vi "取像框架 - 複製.vi"() -> ()   [LabVIEW 2015]
uses:
  <vilib>/userdefined/High Color/IMAQdx.ctl
  <vilib>/vision/driver/NI_Vision_Acquisition_Software.lvlib
  <vilib>/vision/NI_Vision_Development_Module.lvlib
panel:
  in  "開圖":bool
  in  "影像數量":i32=1
  in  "Slide":i16(slide) min=0 scale=0.0..2.0
  in  "Session In":T1="cam1"
  in  "重新開圖":bool
  in  "取像":bool
  out "error out":errorcluster
  in  "stop":bool
  out "Image":T2(plugin-control)
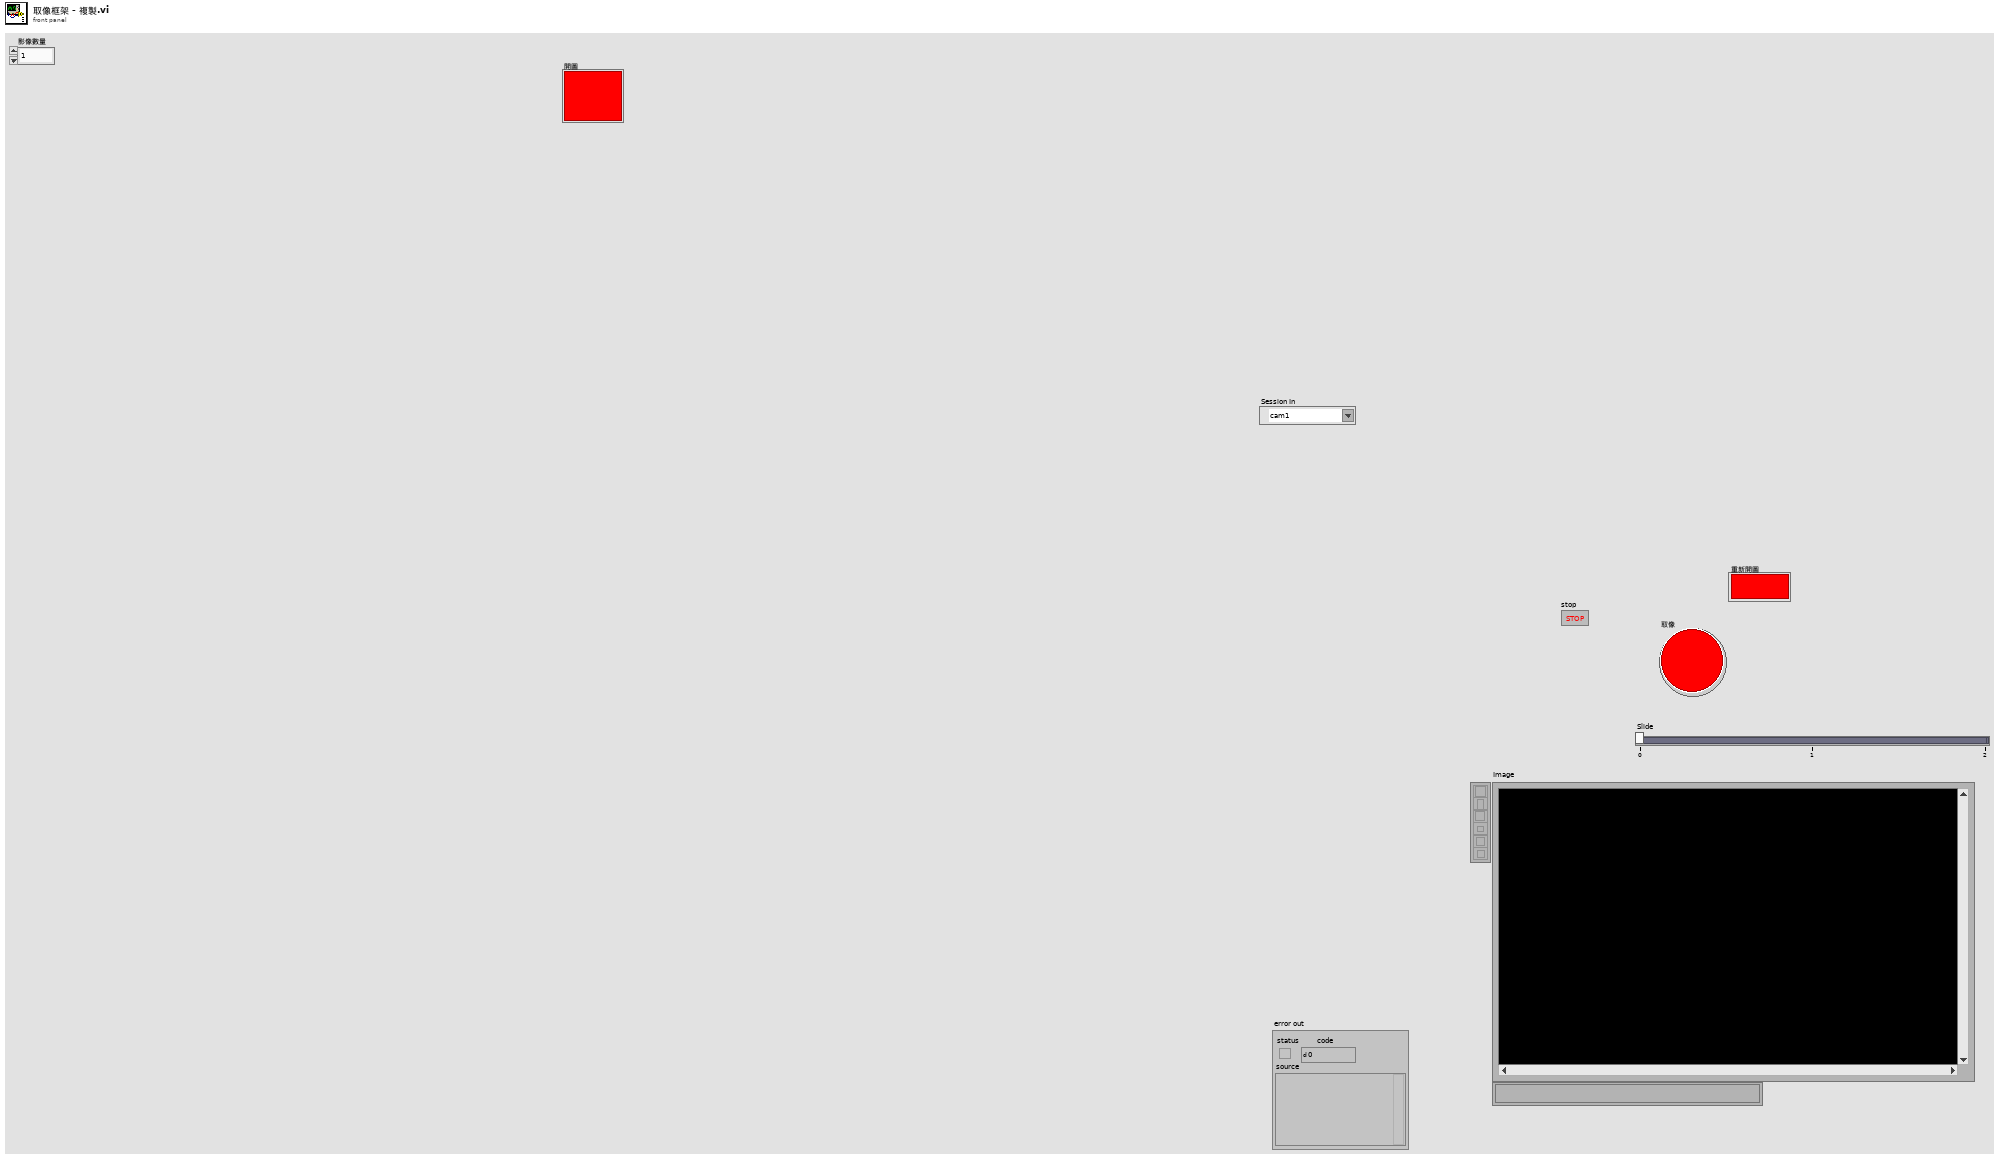
[diagram p1: front panel]
types:
  T1 = typedef "IMAQdx.ctl" = refnum<k21>
  T2 = typedef "IMAQ Image.ctl" = refnum<image>
  T3 = typedef "IMAQ Rectangle" = cluster{"Left":i32, "Top":i32, "Right":i32, "Bottom":i32, "Rotation":dbl}
  T4 = typedef "ROI Descriptor" = cluster{"Global Rectangle":i32[], "Contours":cluster{"ID":enum32{"External", "Internal"}, "Type":u32, "Coordinates":i32[]}[]}
  T5 = cluster{"Global Rectangle":i32[], "Contours":cluster{"Contour Type":u32, "ROI Type":u32, "Points":i32[]}[]}
  T6 = cluster{"Contour Type":u32, "ROI Type":u32, "Points":i32[]}[]
  T7 = cluster{"Contour Type":u32, "ROI Type":u32, "Points":i32[]}
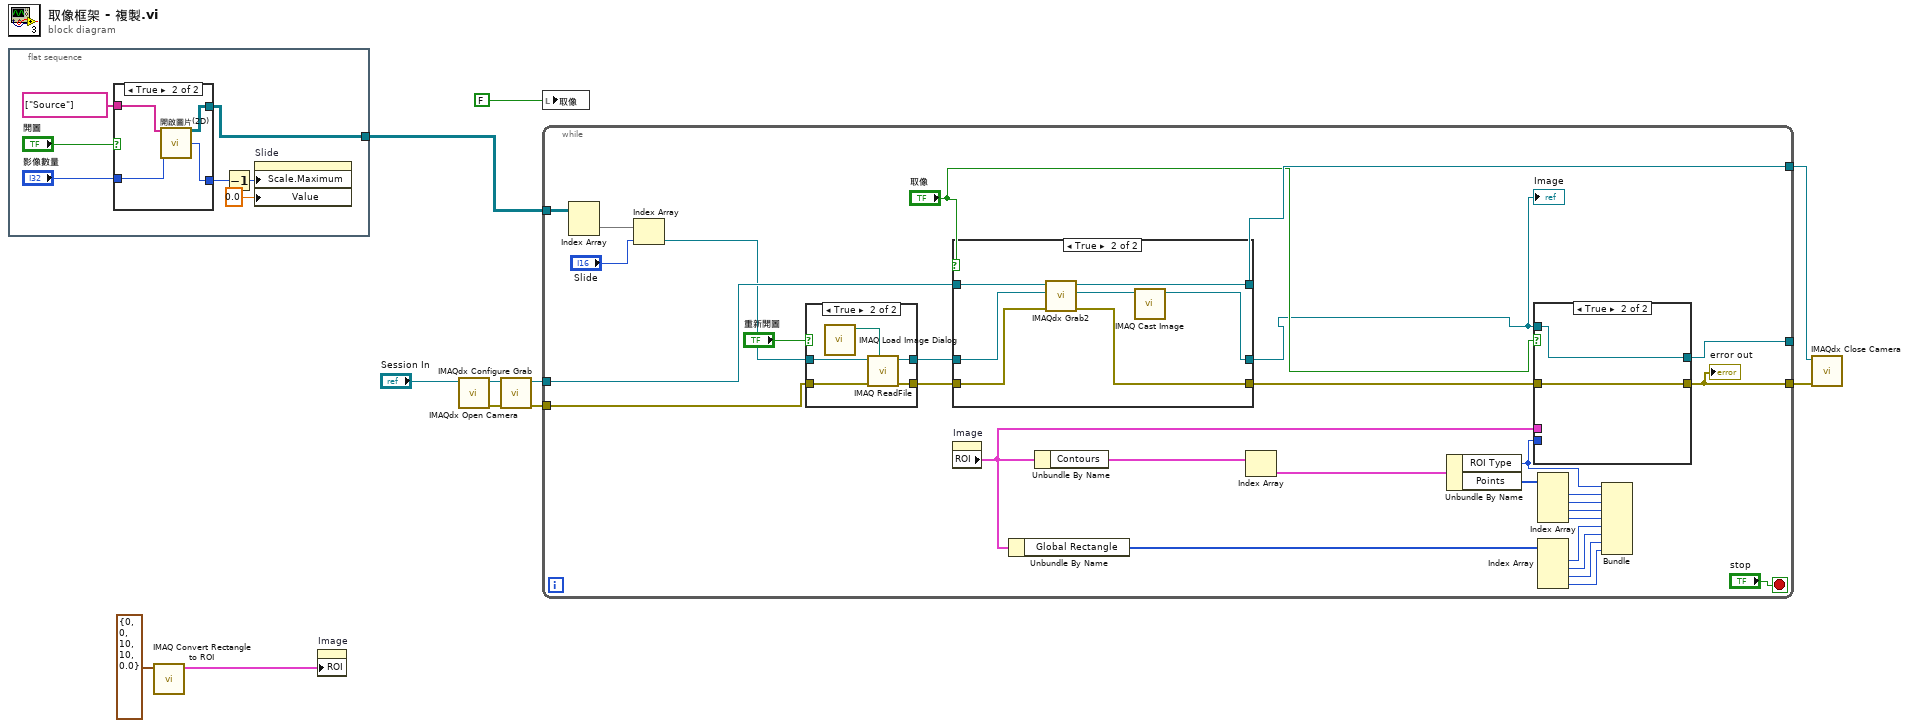
[diagram p0: block diagram]
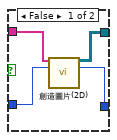
[diagram p2: hidden frame]
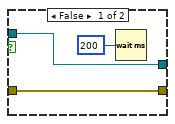
[diagram p4: hidden frame]
diagram:
  n1 = flat-sequence {
    tunnel: [w12] -> w1
    frame #0 {
      n2 = case shown="True" "開圖" {
        tunnel: string[] ["Source"] -> [w20 w26]
        tunnel: [w21 w25] -> w12
        tunnel: [w22 w24] -> w16
        tunnel: "影像數量" -> [w19 w23]
        frame False {
          n3 = call "創造圖片(2D).vi"("ImageNameArray"=w20, "影像數量"=w19) -> ("Image2DArray"=w21:T2[][], "ImageNameNumber"=w22:i32)  [unwired: 10 in, 2 out]
        }
        frame True {
          n4 = call "開啟圖片(2D).vi"("ImageNameArray"=w26, "影像數量"=w23) -> ("Image2DArray"=w25:T2[][], "ImagePathNumber"=w24:i32)  [unwired: 9 in, 3 out]
        }
      }
      n5 = Decrement(x=w16) -> (x-1=w17:i32)
      n6 = property on="Slide" class="Slide (strict)"("Scale.Maximum"=w17, "Value"=0.0 ("Scale.Range:Minimum")) -> ()  [unwired: 2 in, 2 out]
    }
  }
  n7 = call "IMAQ Convert Rectangle to ROI"("Rectangle"=T3 {"Left"=0, "Top"=0, "Right"=10, "Bottom"=10, "Rotation"=0.0}) -> ("ROI Descriptor"=w5:T4)  [unwired: 8 in, 1 out]
  n8 = property on="Image" class="ImageControl"("ROI"=w5) -> ()  [unwired: 2 in, 2 out]
  n9 = call <vilib>:"IMAQdx Open Camera.vi"("Session In"="Session In") -> ("error out"=w7:errorcluster, "Session Out"=w8:T1)  [unwired: 9 in]
  n10 = call <vilib>:"IMAQdx Configure Grab.vi"("error in"=w7, "Session In"=w8) -> ("error out"=w3:errorcluster, "Session Out"=w11:T1)  [unwired: 8 in]
  n11 = local write "取像"(FALSE ("取像")) -> ()
  n12 = while {
    tunnel: w11 -> [w56]
    tunnel: w1 -> [w29]
    tunnel: [w50] -> w10
    tunnel: [w54] -> _
    tunnel: w3 -> [w40]
    tunnel: [w39] -> w2
    stop <- "stop" stop-if-true
    n13 = Index Array(array=w29) -> (element=w30:T2[])  [unwired: 2 in]
    n14 = Index Array(array=w30, index="Slide") -> (element=w28:T2)
    n15 = case shown="True" "重新開圖" {
      tunnel: w28 -> [w58 w61]
      tunnel: [w58 w62] -> w42
      tunnel: w40 -> [w57 w60]
      tunnel: [w57 w59] -> w33
      frame False {
      }
      frame True {
        n16 = call "IMAQ Load Image Dialog"() -> ("Path"=w63:path)  [unwired: 9 in, 2 out]
        n17 = call "IMAQ ReadFile"("File Path"=w63, "error in (no error)"=w60, "Image"=w61) -> ("error out"=w59:errorcluster, "Image Out"=w62:T2)  [unwired: 4 in, 3 out]
      }
    }
    n18 = case shown="True" "取像" {
      tunnel: w56 -> [w71 w78]
      tunnel: w42 -> [w70 w77]
      tunnel: [w71 w76] -> w50
      tunnel: [w70 w73] -> w31
      tunnel: w33 -> [w69 w75]
      tunnel: [w69 w74] -> w41
      frame False {
      }
      frame True {
        n19 = call <vilib>:"IMAQdx Grab2.vi"("error in"=w75, "Image In"=w77, "Session In"=w78) -> ("error out"=w74:errorcluster, "Image Out"=w72:T2, "Session Out"=w76:T1)  [unwired: 5 in, 1 out]
        n20 = call "IMAQ Cast Image"("Image Src"=w72) -> ("Image Dst Out"=w73:T2)  [unwired: 9 in, 1 out]
      }
    }
    "Image" <- w31
    n21 = property on="Image" class="ImageControl"() -> ("ROI"=w49:T5)  [unwired: 2 in, 2 out]
    n22 = Unbundle By Name(w49) -> ("Global Rectangle"=w48:i32[])
    n23 = Unbundle By Name(w49) -> ("Contours"=w53:T6)
    n24 = Index Array(array=w53) -> (element=w52:T7)  [unwired: 1 in]
    n25 = Unbundle By Name(w52) -> ("ROI Type"=w51:u32, "Points"=w38:i32[])
    n26 = case shown="True" "取像" {
      tunnel: w41 -> [w66 w67]
      tunnel: w31 -> [w65 w68]
      tunnel: [w65 w68] -> w54
      tunnel: w49 -> [_ _]
      tunnel: w51 -> [_ _]
      tunnel: [w66 w67] -> w39
      frame False {
        n27 = Wait (ms)(milliseconds to wait=u32 200) -> ()  [unwired: 1 out]
      }
      frame True {
      }
    }
    "error out" <- w39
    n28 = Index Array(array=w38) -> (element #1=w37:i32, element #2=w36:i32, element #3=w34:i32, element #4=w35:i32)  [unwired: 4 in]
    n29 = Index Array(array=w48) -> (element #1=w47:i32, element #2=w46:i32, element #3=w45:i32, element #4=w44:i32)  [unwired: 4 in]
    n30 = Bundle("ROI Type"=w51, w37, w36, w34, w35, w47, w46, w45, w44) -> ()  [unwired: 1 in, 1 out]
  }
  n31 = call <vilib>:"IMAQdx Close Camera.vi"("error in"=w2, "Session In"=w10) -> ()  [unwired: 9 in, 1 out]
